vi "fifoReadHost.vi"() -> ()   [LabVIEW 2017]
uses:
  <vilib>/FPGAPlugInAG/PXI-7852R/niLvFpga_Open_PXI-7852R.vi
  <vilib>/rvi/interface/common/dynamic/niFpgaDynamicAddResources.vi
  <vilib>/Utility/error.llb/Error Cluster From Error Code.vi
  <vilib>/rvi/errors/niLvFpgaAdjustHostInterfaceError.vi
  <vilib>/FPGAPlugInAG/Dynamic/niLvFpga_Close_Dynamic.vi
  <vilib>/rvi/interface/nirviOpenFPGA/nirviOpenFPGA.xnode
  FPGA Bitfiles/PigeonOnFPGA_FPGATarget_analogReadout_ZyKGc9gI8nc.lvbitx
  NI_FPGA/analogReadout.vi
  <vilib>/rvi/interface/nirviMethod/nirviMethod.xnode
  <vilib>/rvi/interface/nirviCloseFPGA/nirviCloseFPGA.xnode
  <vilib>/FPGAPlugInAG/Dynamic/niLvFpga_ReadFifo_Dynamic.vi
  <vilib>/rvi/errors/niLvFpgaMergeErrorWithErrorCode.vi
panel:
  out "Data":i16[](array[numeric])
  out "error out":errorcluster
  in  "stop":bool
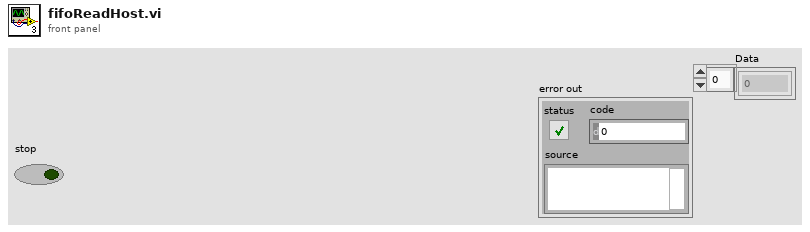
[diagram p1: front panel]
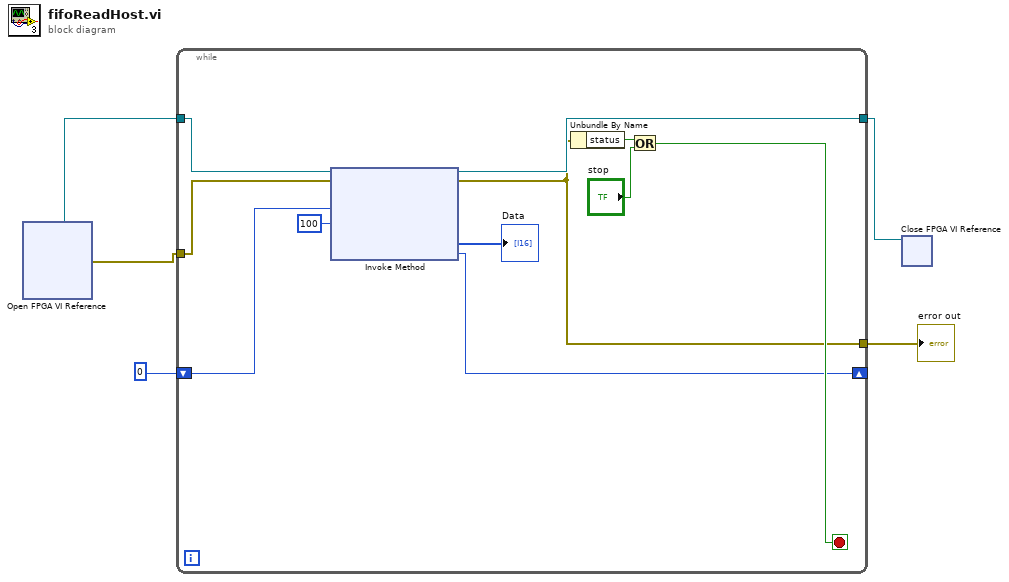
[diagram p0: block diagram]
diagram:
  n1 = xnode "Open FPGA VI Reference"() -> ("FPGA VI Reference Out"=w5:refnum<k20>, "error out"=w4:errorcluster)  [unwired: 2 in]
  n2 = while {
    tunnel: w5 -> [w13]
    tunnel: w4 -> [w11]
    tunnel: [w12] -> w3
    tunnel: [w10] -> w2
    shift-right: [w7] -> _
    shift-left: 0 -> [w8]
    stop <- w14 stop-if-true
    n3 = xnode "Invoke Method"("FPGA VI Reference In"=w13, "error in"=w11, "Number of Elements"=w8, "Timeout (ms)"=100) -> ("FPGA VI Reference Out"=w12:refnum<k20>, "error out"=w10:errorcluster, "Data"=→"Data":i16[], "Elements Remaining"=w7:u32)
    n4 = Unbundle By Name(w10) -> ("status"=w16:bool)
    n5 = Or(x=w16, y="stop") -> (x .or. y?=w14:bool)
  }
  "error out" <- w2
  n6 = xnode "Close FPGA VI Reference"("FPGA VI Reference In"=w3) -> ()  [unwired: 1 in, 1 out]
